vi "Update names group selector.vi"(8 "error in (no error)":errorcluster, 11 "Control-Client in":refnum<class "Control-Client.lvclass">) -> (0 "error out":errorcluster, 3 "Control-Client out":refnum<class "Control-Client.lvclass">)   [LabVIEW 2019, in "Control-Client.lvclass"]
uses:
  Control-Client.lvclass
  Control-Client.lvclass/Control-Client.ctl
  Experiments/Experiments_group.lvclass
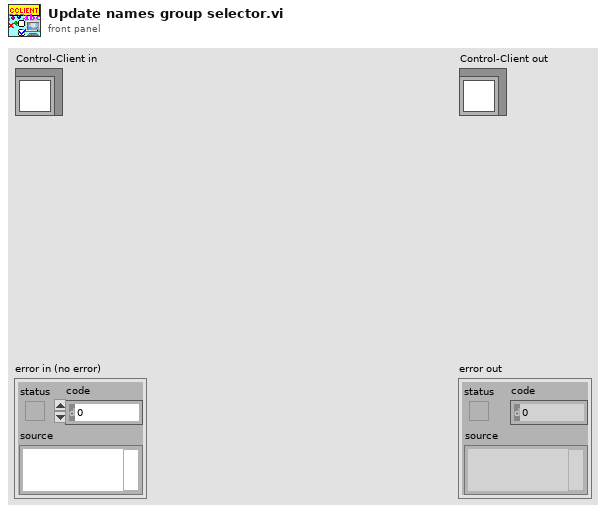
[diagram p1: front panel]
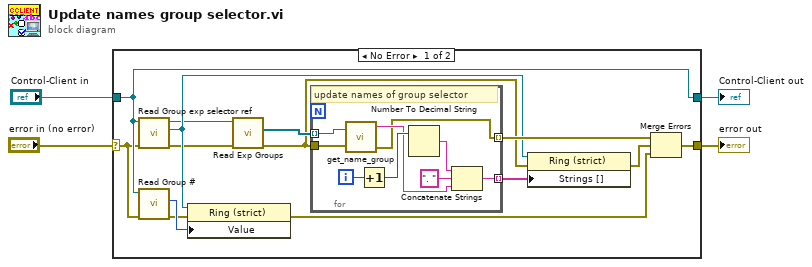
[diagram p0: block diagram]
diagram:
  n1 = case shown="No Error" "error in (no error)" {
    selector: "error in (no error)" -> [w5 w29]
    tunnel: [w15 w29] -> w3
    tunnel: [w6 w28] -> w1
    tunnel: "Control-Client in" -> [w6 w28]
    frame No Error {
      n2 = call "Read Group exp selector ref.vi"("error in (no error)"=w5, "Control-Client in"=w6) -> ("error out"=w8:errorcluster, "Group exp selector ref"=w13:refnum<vi>, "Control-Client out"=w10:refnum<class "Control-Client.lvclass">)  [unwired: 7 in]
      n3 = call "Read Group #.vi"("error in (no error)"=w5, "Control-Client in"=w6) -> ("error out"=w7:errorcluster, "Group #"=w9:i32)  [unwired: 7 in, 1 out]
      n4 = property class="Ring (strict)"(reference=w13, error in=w7, "Value"=w9) -> (error out=w12:errorcluster)  [unwired: 1 out]
      n5 = call "Read Exp Groups.vi"("error in (no error)"=w8, "Control-Client in"=w10) -> ("error out"=w11:errorcluster, "Exp Groups"=w14:refnum<class "Experiments_group.lvclass">[])  [unwired: 7 in, 1 out]
      n6 = for {
        tunnel: [w25] -> w18 mode=indexing
        tunnel: [w21] -> w17 mode=indexing
        tunnel: w14 -> [w20] mode=indexing
        tunnel: w11 -> [w19]
        i -> [w27]
        # "update names of group selector"
        n7 = call-dynamic "get_name_group.vi"("Experiments_group.lvclass in"=w20, "error in (no error)"=w19) -> ("Name"=w22:string, "error out"=w21:errorcluster)  [unwired: 1 out]
        n8 = Increment(x=w27) -> (x+1=w24:i32)
        n9 = Number To Decimal String(number=w24) -> (decimal integer string=w23:string)  [unwired: 1 in]
        n10 = Concatenate Strings(w23, ". " ("string"), w22) -> (w25:string)
      }
      n11 = property on="Property Node" class="Ring (strict)"(reference=w13, error in=w11, "Strings []"=w18) -> (error out=w16:errorcluster)  [unwired: 1 out]
      n12 = Merge Errors(w17, w16, w12) -> (w15:errorcluster)
    }
    frame Error {
    }
  }
  "error out" <- w3
  "Control-Client out" <- w1
